vi "Initialize Bus Controller.vi"(8 "error in":errorcluster, 11 "module handle":u32) -> (0 "error out":errorcluster, 3 "module handle out":u32)   [LabVIEW 2020, in "AIM MIL-STD-1553 Hardware API.lvlib"]
doc: "Used to create a single transfer, including associated headers and data buffers.\n\n<B>Input Parameters:</B>\n\nModule Handle - Reference to the device as obtained from a call to: 1553 General - Obtain a Device Reference.vi\n\nData Array (32 words, all zero) - The input data array for the buffer.\n\n<B>BC Transfer Descriptor:</B>\n\nTransfer ID - The ID number of the transfer to define.\n\nTransfer Type - The type of transfer to define (BC to RT, RT to BC,...).\n\nBus - The bus on which the transfer will initially be sent (primary, secondary).\n\nTransmitting RT Address - Address of the transmitter (ignored for BC->RT transfers). Set to 31 for broadcast.\n\nReceiving RT Address - Address of the receiver (ignored for RT->BC transfers). Set to 32 for broadcast.\n\nTransmitting RT Sub-address - Address of the transmitter (ignored for BC->RT transfers). Set to 0, 31 for mode codes.\n\nReceiving RT Sub-address - Address of the receiver (ignored for RT->BC transfers). Set to 0, 31 for mode codes.\n\nWord Count / Mode Code - Word count / mode code for the transfer. Use 0 for 32 words. All others (1.. 31) are the actual word count.\n\nGap Mode - The gap timing mode for this transferr. Possible values are: \n\ndelay -\n In this mode, the Transfer Wait Time specifies the time from the start of a transfer to the start of the following transfer in microseconds. Note that if the specified time is shorter than the actual time needed for transfer transmission, the Transfer Wait Time is ignored and the bus controller automatically generates a minimum intermessage gap of approximately 11 microseconds. This gap mode guarantees deterministic framing independent from RT response times and provides excellent repeatability of timed bus events. In this mode, Transfer Wait Time is in units of microseconds.\n\nstandard - \n In standard gap mode, the Transfer Wait Time specifies the wait gap between the end of the current transfer and start of the following transmitted command word. The nominal intermessage gap time is given by the Transfer Wait Time in microseconds. Note that the idle time of the physical bus is 2 microseconds less than this time due to the gap measurement definition of MIL-STD-1553B. Also note that the minimum intermessage gap time achieved using the standard gap mode is equal to the minimum gap time achieved in the Transfer Wait Time mode. Finally, note that for broadcast transfers, the response timeout is used to check that no status word is responded. Thus, the intermessage gap time in standard mode shall be greater than the response timeout, to guarantee proper operation.\n\nfast - \n In the fast gap mode, the bus controller generates intermessage gap times down to 4 microseconds. In this mode, the value of the Transfer Wait Time is limited to 6 bits. The nominal intermessage gap time is calculated as: 4 microseconds + (Transfer Wait Time * 0.25 microseconds). \n Therefore, intermessage gap times between 4 microseconds, and up to 19.75 microseconds can be achieved in this mode. This mode can be used for RT validation and testing, but shall not be used during normal operation since line busy and word count high checks are disabled on the BC. Also worst case operation is not guaranteed if this mode is combined with Multi RT, monitor and mailbox operation.\n The Fast Gap Mode shall only be used for transfer instructions which are followed by another transfer instruction. In case of a transfer error, the Fast Gap Mode is switched off for this transfer and a default Intermessage gap of approximately 11 microseconds is generated.\n\nTransfer Wait Time - Refer to the description of the gap modes (above) for possible values.\n\n<B>Transfer Options (none):</B>\n\nInterrupt Control - Interrupt control mode for the transfer. Possible values are: none, on end of transfer, on transfer error, on status word exception.\n\nHalt Control - Halt on exception control mode for the transfer. Possible values are: none, on transfer error, on status word exception, on both [transfer error and status word exception], on any interrupt.\n\nRetry Control - Retry control mode for the transfer. Possible values are: disable, enable, keep bus at next transmit, alternate bus on next transmit.\n\nExpected Response - Response expected as a result of the transfer. Possible values are: automatic, no status word 1, no status word 2.\n\n<B>Error Injection (none):</B>\n\nError Type - The type of error to inject. This can be one of the following values:\n\nnone -\n Perform no error injection.\n\ncommand synch error -\n Command sync eror with the sync pattern in Synch Field Error.\n\ndata synch error -\n Data sync error with sync pattern in Synch Field Error, in the word given in Word Position.\n\nparity error -\n Parity error in the word given in Word Position.\n\nManchester bit stuck on high -\nManchester bit stuck on low -\n Manchester encoding error such that the bit given in Bit Position, in the word given in Word Position is stuck on either high or low.\n\ngap error -\n Gap error with the gap defined in Gap/Zero Crossing, in the word given in Word Position.\n\nword count too high -\nword count too low -\n Word count too high or too low, with the erronious count given in Word Position.\n\nbit count too high -\nbit count too low -\n Bit count too high or too low, for the word given in Word Position. For the too high error, the value of the bit count will be the actual count + Bit Count. For the too low error, the value will be the actual - Bit Count. Bit count errors are not supported for mode code transfers without data.\n\nzero crossing low deviation -\nzero crossing high deviation -\n Zero crossing low or high deviation error in the word given in Word Position, at the bit given in Bit Position, and with negative or positive deviation in Gap/Zero Crossing.\n\nbus switching support -\n The BIU disables the physical decoder device on the alternate bus, if the current transfer is in fast gap mode (used for RT-Validation Test 5.2.1.8).\n\n<B> Output Parameters: </B>\n\nTransfer ID out - A copy of the original transfer ID that was assigned."
uses:
  AIM MIL-STD-1553 Hardware API.lvlib
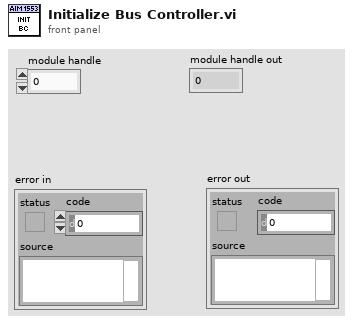
[diagram p1: front panel]
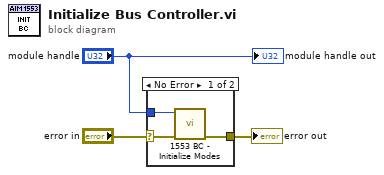
[diagram p0: block diagram]
diagram:
  n1 = case shown="No Error" "error in" {
    selector: "error in" -> [w6 w7]
    tunnel: [w5 w7] -> w2
    tunnel: "module handle" -> [w4 _]
    frame No Error {
      n2 = call <instrlib>:"1553 BC - Initialize Modes.vi"("Error In (none)"=w6, "Module Handle"=w4) -> ("Error Out"=w5:errorcluster)  [unwired: 9 in]
    }
    frame Error {
    }
  }
  "error out" <- w2
  "module handle out" <- "module handle"
